vi "Calcula_Proteção.vi"(5 "Zenital angle rad":dbl, 6 "Azimute rad":dbl) -> (0 "Z_SEGURANÇA_GRAUS":dbl, 1 "Prot Segur":bool, 2 "Z_LIBERA_GRAUS":dbl, 3 "Z_MAX_GRAUS":dbl, 4 "Prot Zmax":bool)   [LabVIEW 2018]
uses:
  Global_Telescopio.vi
panel:
  out "Numeric":i32
  out "libera":dbl
  out "segur":dbl
  out "max":dbl
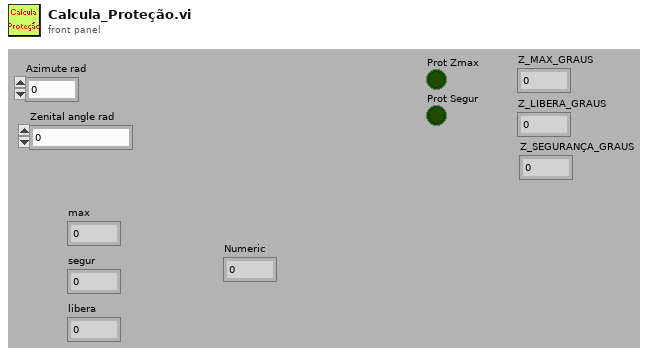
[diagram p1: front panel]
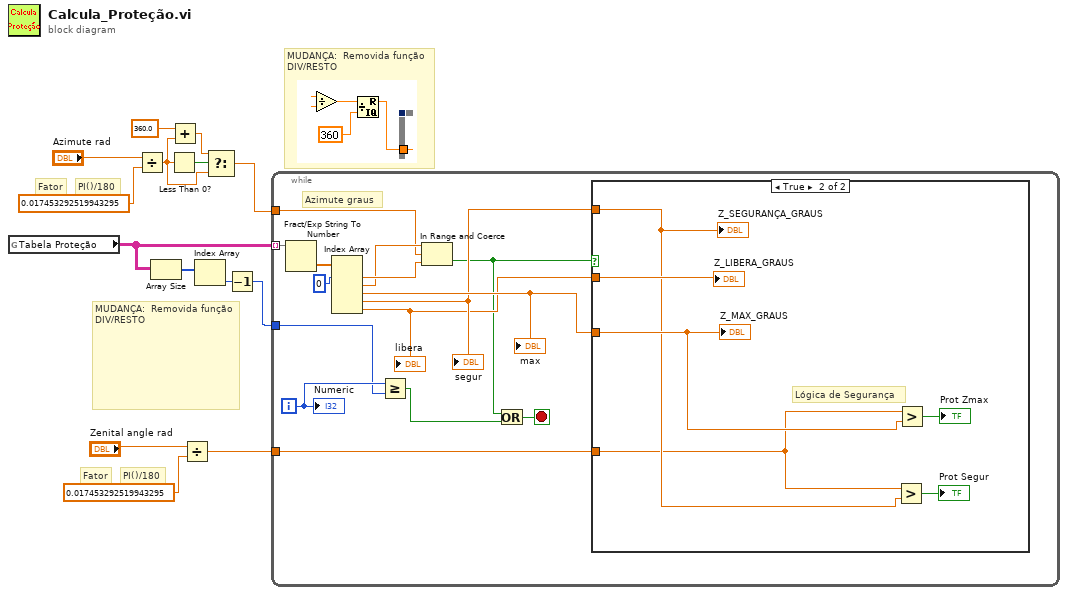
[diagram p0: block diagram]
diagram:
  # "MUDANÇA:  Removida função \nDIV/RESTO"
  # "MUDANÇA:  Removida função \nDIV/RESTO"
  # "Fator"
  # "PI()/180"
  # "Fator"
  # "PI()/180"
  n1 = global read "Global_Telescopio.vi" "Tabela Proteção"() -> (w14:string[][])
  n2 = Divide(x="Azimute rad", y=0.017453292519943295) -> (x/y=w1:dbl)
  n3 = Array Size(array=w14) -> (size(s)=w13:i32[])
  n4 = Less Than 0?(x=w1) -> (x < 0?=w5:bool)
  n5 = Add(x=360.0, y=w1) -> (x+y=w3:dbl)
  n6 = Divide(x="Zenital angle rad", y=0.017453292519943295) -> (x/y=w6:dbl)
  n7 = Index Array(array=w13) -> (element=w12:i32)  [unwired: 1 in]
  n8 = Select(t=w3, s=w5, f=w1) -> (s? t:f=w4:dbl)
  n9 = Decrement(x=w12) -> (x-1=w11:i32)
  n10 = while {
    tunnel: w14 -> [w29] mode=indexing
    tunnel: w11 -> [w21]
    tunnel: w4 -> [w16]
    tunnel: w6 -> [w15]
    i -> [w22]
    stop <- w24 stop-if-true
    # "Azimute graus"
    n11 = Fract/Exp String To Number(string=w29) -> (number=w28:dbl[])  [unwired: 3 in, 1 out]
    n12 = Index Array(array=w28, index #1=0 ("index")) -> (element #1=w26:dbl, element #2=w25:dbl, element #3=w20:dbl, element #4=w19:dbl, element #5=w18:dbl)  [unwired: 4 in]
    "max" <- w20
    "segur" <- w19
    "libera" <- w18
    n13 = Greater Or Equal?(x=w22, y=w21) -> (x >= y?=w23:bool)
    n14 = In Range and Coerce(upper limit=w25, x=w16, lower limit=w26) -> (In Range?=w17:bool)  [unwired: 1 out]
    n15 = Or(x=w17, y=w23) -> (x .or. y?=w24:bool)
    n16 = case shown="True" w17 {
      tunnel: w20 -> [_ w34]
      tunnel: w19 -> [_ w33]
      tunnel: w18 -> [_ w35]
      tunnel: w15 -> [_ w30]
      frame False {
      }
      frame True {
        # "Lógica de Segurança"
        n17 = Greater?(x=w30, y=w33) -> (0:→"Prot Segur":bool)
        n18 = Greater?(x=w30, y=w34) -> (0:→"Prot Zmax":bool)
        "Z_SEGURANÇA_GRAUS" <- w33
        "Z_LIBERA_GRAUS" <- w35
        "Z_MAX_GRAUS" <- w34
      }
    }
    "Numeric" <- w22
  }
